vi "defendAreaTacticCheckStateChange.vi"(8 "error in (no error)":errorcluster, 11 "DefendAreaTacticVSS in":refnum<class "DefendAreaTacticVSS.lvclass">) -> (0 "error out":errorcluster, 2 "State":enum16{"Exit", "Kick", "DefBallPos", "GoToBall"}(ring), 3 "DefendAreaTacticVSS out":refnum<class "DefendAreaTacticVSS.lvclass">)   [LabVIEW 2020, in "DefendAreaTacticVSS.lvclass"]
uses:
  DefendAreaTacticVSS.lvclass
  Game_class/Game.lvclass
  Robot_class/Robot.lvclass
  Utilities_class/Utilities.lvclass
  Game_class/Game.lvclass/Game.ctl
  Object_class/Object.lvclass/Object.ctl
  Team_class/Team.lvclass/Team.ctl
  Events_class/Events.lvclass/Events.ctl
  Object_class/Read x.vi
  Object_class/Read y.vi
  Game_class/Read BallRef.vi
  Game_class/Read EnemyRef.vi
  Game_class/Read EventsRef.vi
  Events_class/Read id_touch.vi
  Team_class/Read RobotRef.vi
  Enemy_class/Enemy.lvclass
  Ball_class/Ball.lvclass
  Events_class/Events.lvclass
panel:
  in  "Robot In":refnum<class "Robot.lvclass">
  in  "Game in":refnum<class "Game.lvclass">
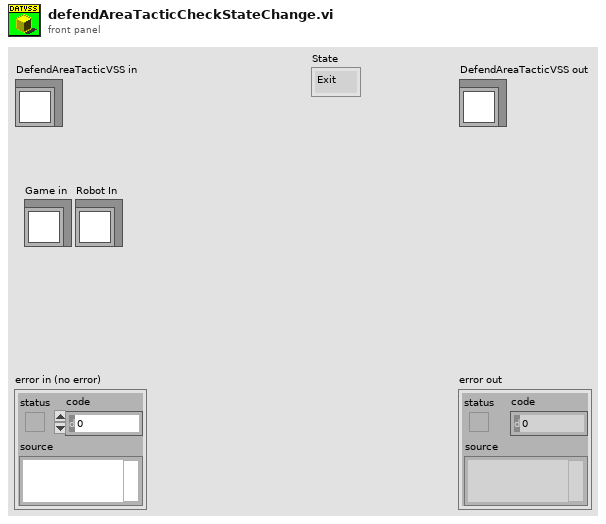
[diagram p1: front panel]
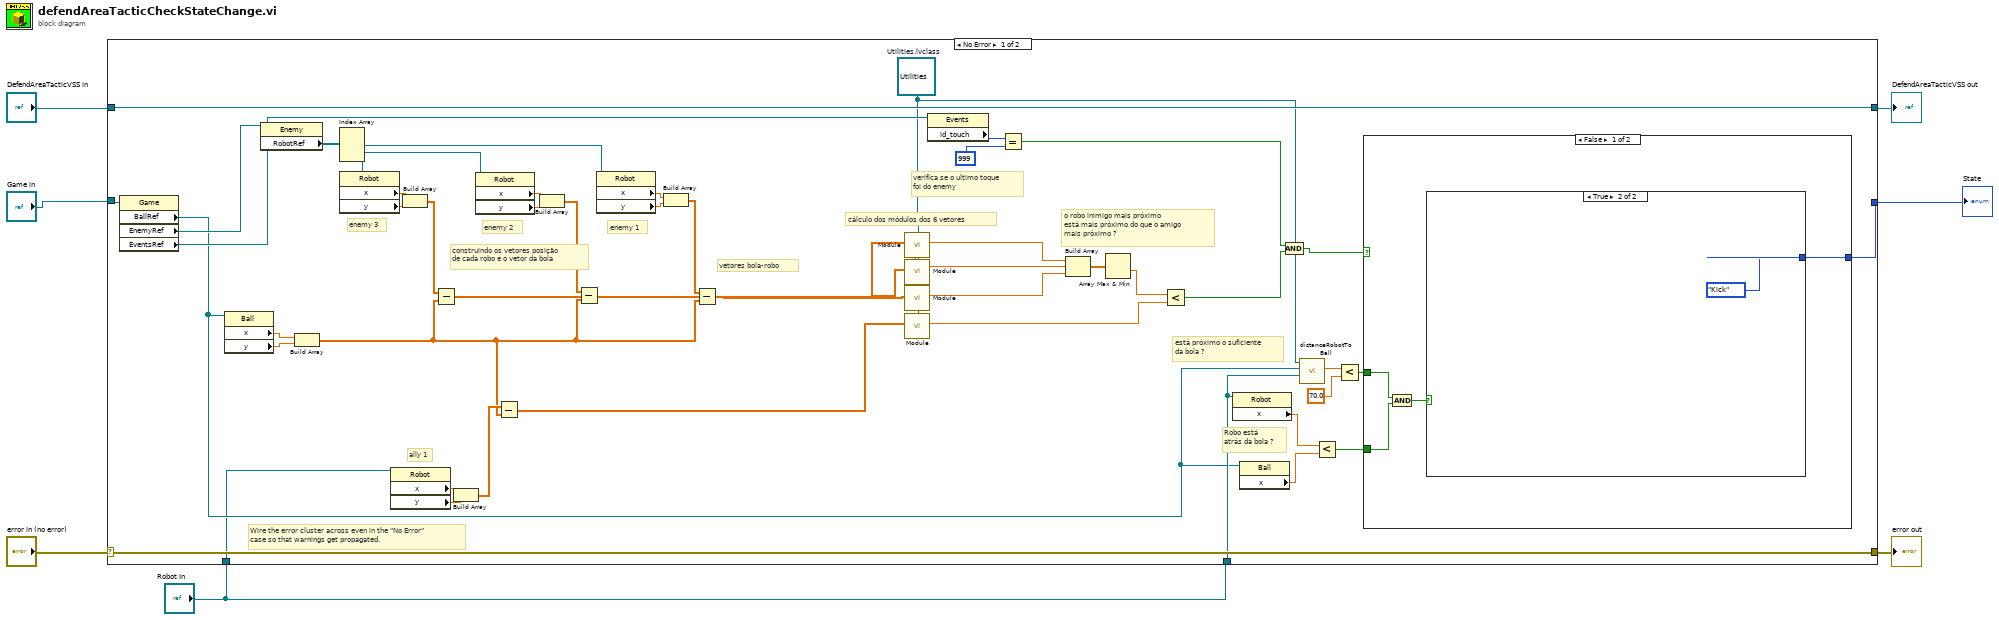
[diagram p0: block diagram]
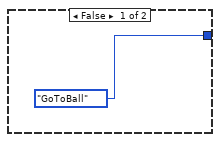
[diagram p2: hidden frame]
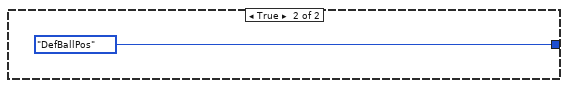
[diagram p3: hidden frame]
diagram:
  n1 = case shown="No Error" "error in (no error)" {
    selector: "error in (no error)" -> [w56 w66]
    tunnel: [w56 w66] -> w6
    tunnel: [w57 w65] -> w4
    tunnel: "DefendAreaTacticVSS in" -> [w57 w65]
    tunnel: [w20 _] -> w3
    tunnel: "Game in" -> [w55 _]
    tunnel: "Robot In" -> [w15 _]
    tunnel: "Robot In" -> [w9 _]
    frame No Error {
      w16 = refnum<class "Utilities.lvclass"> refnum  # Utilities.lvclass
      # "está próximo o suficiente\nda bola ?"
      # "Robo está\natrás da bola ?"
      # "o robo inimigo mais próximo\nestá mais próximo do que o amigo\nmais próximo ?"
      # "cálculo dos módulos dos 6 vetores"
      # "vetores bola-robo"
      # "verifica se o ultimo toque\nfoi do enemy"
      # "construindo os vetores posição \nde cada robo e o vetor da bola"
      # "ally 1"
      # "enemy 1"
      # "enemy 2"
      # "enemy 3"
      # "Wire the error cluster across even in the \"No Error\"\ncase so that warnings get propagated."
      n2 = property class="Game"(reference=w55) -> ("BallRef"=w14:refnum<class "Ball.lvclass">, "EnemyRef"=w54:refnum<class "Enemy.lvclass">, "EventsRef"=w49:refnum<class "Events.lvclass">)  [unwired: 1 in, 2 out]
      n3 = property class="Ball"(reference=w14) -> ("x"=w45:dbl, "y"=w44:dbl)  [unwired: 1 in, 2 out]
      n4 = property class="Enemy"(reference=w54) -> ("RobotRef"=w53:refnum<class "Robot.lvclass">[])  [unwired: 1 in, 2 out]
      n5 = Build Array(w45, w44) -> (w31:dbl[])
      n6 = Index Array(array=w53) -> (element #1=w52:refnum<class "Robot.lvclass">, element #2=w51:refnum<class "Robot.lvclass">, element #3=w50:refnum<class "Robot.lvclass">)  [unwired: 3 in]
      n7 = property class="Robot"(reference=w50) -> ("x"=w43:dbl, "y"=w42:dbl)  [unwired: 1 in, 2 out]
      n8 = property class="Robot"(reference=w9) -> ("x"=w37:dbl, "y"=w36:dbl)  [unwired: 1 in, 2 out]
      n9 = Build Array(w43, w42) -> (w35:dbl[])
      n10 = Subtract(x=w35, y=w31) -> (x-y=w30:dbl[])
      n11 = Build Array(w37, w36) -> (w32:dbl[])
      n12 = property class="Robot"(reference=w51) -> ("x"=w41:dbl, "y"=w40:dbl)  [unwired: 1 in, 2 out]
      n13 = Subtract(x=w32, y=w31) -> (x-y=w27:dbl[])
      n14 = Build Array(w41, w40) -> (w34:dbl[])
      n15 = Subtract(x=w34, y=w31) -> (x-y=w29:dbl[])
      n16 = property class="Robot"(reference=w52) -> ("x"=w39:dbl, "y"=w38:dbl)  [unwired: 1 in, 2 out]
      n17 = Build Array(w39, w38) -> (w33:dbl[])
      n18 = Subtract(x=w33, y=w31) -> (x-y=w28:dbl[])
      n19 = call-dynamic "Module.vi"("2D vector"=w30, "Utilities in"=w16) -> ("Modulo"=w26:dbl)  [unwired: 7 in, 2 out]
      n20 = call-dynamic "Module.vi"("2D vector"=w29, "Utilities in"=w16) -> ("Modulo"=w25:dbl)  [unwired: 7 in, 2 out]
      n21 = call-dynamic "Module.vi"("2D vector"=w28, "Utilities in"=w16) -> ("Modulo"=w24:dbl)  [unwired: 7 in, 2 out]
      n22 = call-dynamic "Module.vi"("2D vector"=w27, "Utilities in"=w16) -> ("Modulo"=w8:dbl)  [unwired: 7 in, 2 out]
      n23 = property class="Events"(reference=w49) -> ("id_touch"=w48:i32)  [unwired: 1 in, 2 out]
      n24 = Equal?(x=w48, y=999) -> (x = y?=w22:bool)
      n25 = Build Array(w26, w25, w24) -> (w46:dbl[])
      n26 = Array Max & Min(array=w46) -> (min value=w23:dbl)  [unwired: 3 out]
      n27 = Less?(x=w23, y=w8) -> (x < y?=w21:bool)
      n28 = property class="Robot"(reference=w15) -> ("x"=w18:dbl)  [unwired: 1 in, 2 out]
      n29 = property class="Ball"(reference=w14) -> ("x"=w17:dbl)  [unwired: 1 in, 2 out]
      n30 = And(x=w22, y=w21) -> (x .and. y?=w19:bool)
      n31 = call "distanceRobotToBall.vi"("Robot"=w15, "Ball"=w14, "Utilities in"=w16) -> ("Distance Robot To Ball"=w12:dbl)  [unwired: 6 in, 2 out]
      n32 = Less?(x=w18, y=w17) -> (x < y?=w10:bool)
      n33 = Less?(x=w12, y=70.0) -> (x < y?=w11:bool)
      n34 = case shown="False" w19 {
        tunnel: [w61 enum16{"Exit", "Kick", "DefBallPos", "GoToBall"}."DefBallPos" ("State")] -> w20
        tunnel: w11 -> [w60 _]
        tunnel: w10 -> [w59 _]
        frame False {
          n35 = And(x=w60, y=w59) -> (x .and. y?=w58:bool)
          n36 = case shown="True" w58 {
            tunnel: [enum16{"Exit", "Kick", "DefBallPos", "GoToBall"}."GoToBall" ("State") enum16{"Exit", "Kick", "DefBallPos", "GoToBall"}."Kick" ("State")] -> w61
            frame False {
            }
            frame True {
            }
          }
        }
        frame True {
        }
      }
    }
    frame Error {
    }
  }
  "error out" <- w6
  "DefendAreaTacticVSS out" <- w4
  "State" <- w3
